vi "HexStringToBase64.vi"(1 "Hex":string) -> (0 "BASE64 string":string)   [LabVIEW 2023]
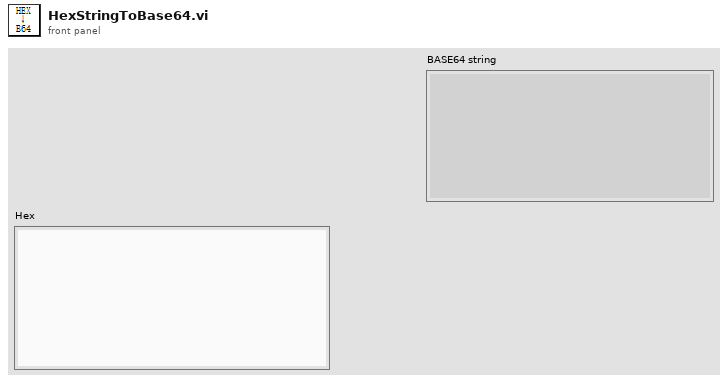
[diagram p1: front panel]
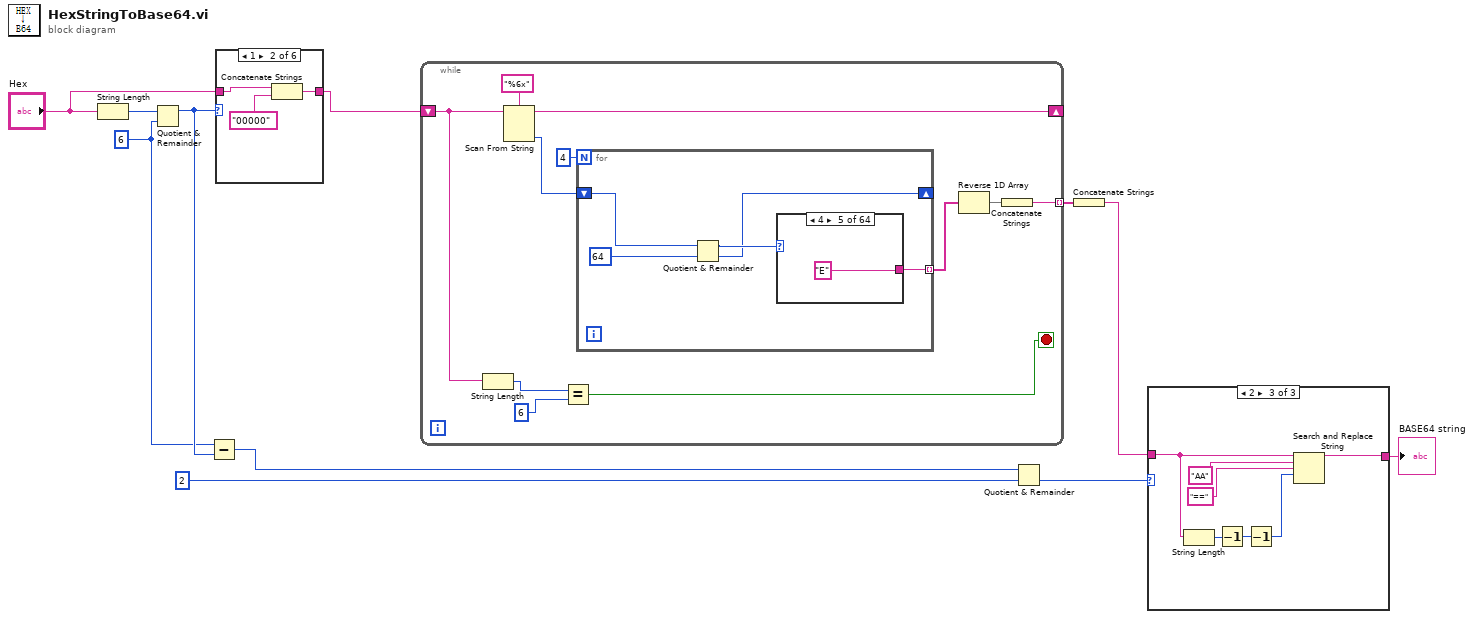
[diagram p0: block diagram]
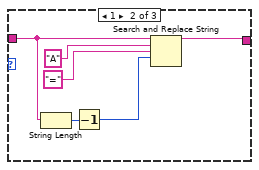
[diagram p3: hidden frame]
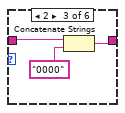
[diagram p5: hidden frame]
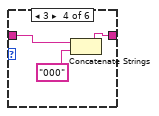
[diagram p6: hidden frame]
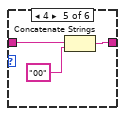
[diagram p7: hidden frame]
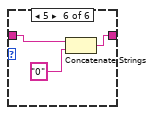
[diagram p8: hidden frame]
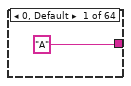
[diagram p9: hidden frame]
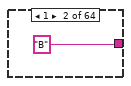
[diagram p10: hidden frame]
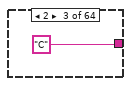
[diagram p11: hidden frame]
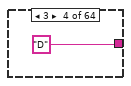
[diagram p12: hidden frame]
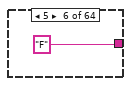
[diagram p13: hidden frame]
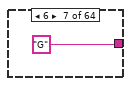
[diagram p14: hidden frame]
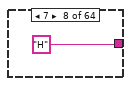
[diagram p15: hidden frame]
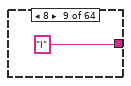
[diagram p16: hidden frame]
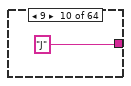
[diagram p17: hidden frame]
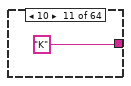
[diagram p18: hidden frame]
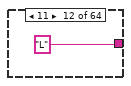
[diagram p19: hidden frame]
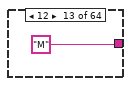
[diagram p20: hidden frame]
diagram:
  w4 = u64 6
  n1 = String Length(string="Hex") -> (length=w11:i32)
  n2 = Quotient & Remainder(x=w11, y=w4) -> (x-y*floor(x/y)=w5:u64)  [unwired: 1 out]
  n3 = Subtract(x=w4, y=w5) -> (x-y=w6:u64)
  n4 = case shown="1" w5 {
    tunnel: [w12 w15 w16 w19 w22 w25] -> w9
    tunnel: "Hex" -> [w12 w14 w17 w20 w23 w26]
    frame 0, Default {
    }
    frame 1 {
      n5 = Concatenate Strings(w14, "00000") -> (w15:string)
    }
    frame 2 {
      n6 = Concatenate Strings(w17, "0000") -> (w16:string)
    }
    frame 3 {
      n7 = Concatenate Strings(w20, "000") -> (w19:string)
    }
    frame 4 {
      n8 = Concatenate Strings(w23, "00") -> (w22:string)
    }
    frame 5 {
      n9 = Concatenate Strings(w26, "0") -> (w25:string)
    }
  }
  n10 = while {
    shift-right: [w38] -> _
    shift-left: w9 -> [w33]
    tunnel: [w28] -> w8 mode=indexing
    stop <- w31 stop-if-true
    n11 = String Length(string=w33) -> (length=w32:i32)
    n12 = Scan From String(format string="%6x", input string=w33) -> (remaining string=w38:string, output 1=w36:u32)  [unwired: 3 in, 2 out]
    n13 = Equal?(x=w32, y=6) -> (x = y?=w31:bool)
    n14 = for {
      N: 4 -> [_]
      tunnel: [w43] -> w30 mode=indexing
      shift-right: [w39] -> _
      shift-left: w36 -> [w42]
      n15 = Quotient & Remainder(x=w42, y=u64 64) -> (x-y*floor(x/y)=w40:u64, floor(x/y)=w39:u64)
      n16 = case shown="4" w40 {
        tunnel: ["A" "B" "C" "D" "E" "F" "G" "H" "I" "J" "K" "L" "M" "N" "O" "P" "Q" "R" "S" "T" "U" "V" "W" "X" "Y" "Z" "a" "b" "c" "d" "e" "f" "g" "h" "i" "j" "k" "l" "m" "n" "o" "p" "q" "r" "s" "t" "u" "v" "w" "x" "y" "z" "0" "1" "2" "3" "4" "5" "6" "7" "8" "9" "+" "/"] -> w43
        frame 0, Default {
        }
        frame 1 {
        }
        frame 2 {
        }
        frame 3 {
        }
        frame 4 {
        }
        frame 5 {
        }
        frame 6 {
        }
        frame 7 {
        }
        frame 8 {
        }
        frame 9 {
        }
        frame 10 {
        }
        frame 11 {
        }
        frame 12 {
        }
        frame 13 {
        }
        frame 14 {
        }
        frame 15 {
        }
        frame 16 {
        }
        frame 17 {
        }
        frame 18 {
        }
        frame 19 {
        }
        frame 20 {
        }
        frame 21 {
        }
        frame 22 {
        }
        frame 23 {
        }
        frame 24 {
        }
        frame 25 {
        }
        frame 26 {
        }
        frame 27 {
        }
        frame 28 {
        }
        frame 29 {
        }
        frame 30 {
        }
        frame 31 {
        }
        frame 32 {
        }
        frame 33 {
        }
        frame 34 {
        }
        frame 35 {
        }
        frame 36 {
        }
        frame 37 {
        }
        frame 38 {
        }
        frame 39 {
        }
        frame 40 {
        }
        frame 41 {
        }
        frame 42 {
        }
        frame 43 {
        }
        frame 44 {
        }
        frame 45 {
        }
        frame 46 {
        }
        frame 47 {
        }
        frame 48 {
        }
        frame 49 {
        }
        frame 50 {
        }
        frame 51 {
        }
        frame 52 {
        }
        frame 53 {
        }
        frame 54 {
        }
        frame 55 {
        }
        frame 56 {
        }
        frame 57 {
        }
        frame 58 {
        }
        frame 59 {
        }
        frame 60 {
        }
        frame 61 {
        }
        frame 62 {
        }
        frame 63 {
        }
      }
    }
    n17 = Reverse 1D Array(array=w30) -> (reversed array=w29:string[])
    n18 = Concatenate Strings(w29) -> (w28:string)
  }
  n19 = Quotient & Remainder(x=w6, y=2) -> (floor(x/y)=w3:u64)  [unwired: 1 out]
  n20 = Concatenate Strings(w8) -> (w2:string)
  n21 = case shown="2" w3 {
    tunnel: w2 -> [w108 w110 w117]
    tunnel: [w108 w109 w116] -> w1
    frame 0, Default {
    }
    frame 1 {
      n22 = String Length(string=w110) -> (length=w112:i32)
      n23 = Decrement(x=w112) -> (x-1=w111:i32)
      n24 = Search and Replace String(input string=w110, search string="A", replace string="=", offset=w111) -> (result string=w109:string)  [unwired: 4 in, 3 out]
    }
    frame 2 {
      n25 = String Length(string=w117) -> (length=w119:i32)
      n26 = Decrement(x=w119) -> (x-1=w118:i32)
      n27 = Decrement(x=w118) -> (x-1=w115:i32)
      n28 = Search and Replace String(input string=w117, search string="AA", replace string="==", offset=w115) -> (result string=w116:string)  [unwired: 4 in, 3 out]
    }
  }
  "BASE64 string" <- w1
